vi "Add State to Queue.vi"(0 "State(s) In Front (\"\")":string, 5 "State(s) In (\"\")":string, 7 "State(s) At Back (\"\")":string) -> (6 "States Out":string)   [LabVIEW 2016, in "斯坦道氨氮V2.lvlib"]
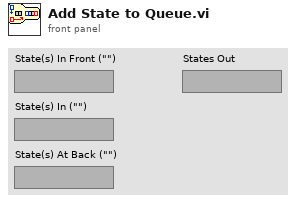
[diagram p1: front panel]
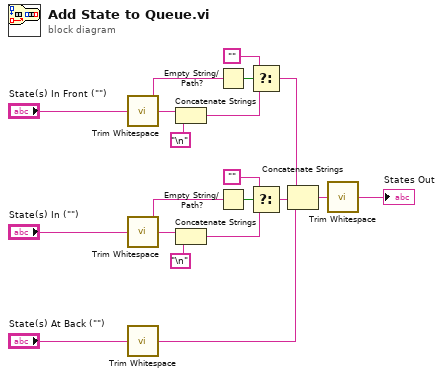
[diagram p0: block diagram]
diagram:
  n1 = call <vilib>:"Trim Whitespace.vi"("string"="State(s) In Front (\"\")") -> ("trimmed string"=w14:string)  [unwired: 1 in]
  n2 = call <vilib>:"Trim Whitespace.vi"("string"="State(s) In (\"\")") -> ("trimmed string"=w13:string)  [unwired: 1 in]
  n3 = call <vilib>:"Trim Whitespace.vi"("string"="State(s) At Back (\"\")") -> ("trimmed string"=w1:string)  [unwired: 1 in]
  n4 = Concatenate Strings(w14, "\n") -> (w16:string)
  n5 = Concatenate Strings(w13, "\n") -> (w11:string)
  n6 = Empty String/Path?(string/path=w14) -> (empty?=w18:bool)
  n7 = Empty String/Path?(string/path=w13) -> (empty?=w9:bool)
  n8 = Select(t="", s=w18, f=w16) -> (s? t:f=w7:string)
  n9 = Select(t="", s=w9, f=w11) -> (s? t:f=w8:string)
  n10 = Concatenate Strings(w7, w8, w1) -> (w5:string)
  n11 = call <vilib>:"Trim Whitespace.vi"("string"=w5) -> ("trimmed string"=→"States Out":string)  [unwired: 1 in]
